vi "Build HW Tree.vi"(8 "error in (no error)":errorcluster, 10 "HW Info":T1[](array[typedef]), 11 "Hardware Info Module in":refnum<class "Hardware Info Module.lvclass">) -> (0 "error out":errorcluster, 3 "Hardware Info Module out":refnum<class "Hardware Info Module.lvclass">)   [LabVIEW 2023, in "Volatus.lvlib" / "Hardware Info Module.lvclass"]
uses:
  Hardware Info Module.lvclass
  HW Info.ctl
  lv-cdm/CDM-Config/Config-JSON/Config-JSON.lvclass
  Hardware Info Module.lvclass/Hardware Info Module.ctl
  lv-cdm/CDM-Config/Config Element/Config Element.lvclass
  lv-cdm/CDM-Config/Config Manager/Config Manager.lvclass
  <vilib>/JDP Science/JSONtext/JSONtext.lvlib
panel:
  out "JSON":string
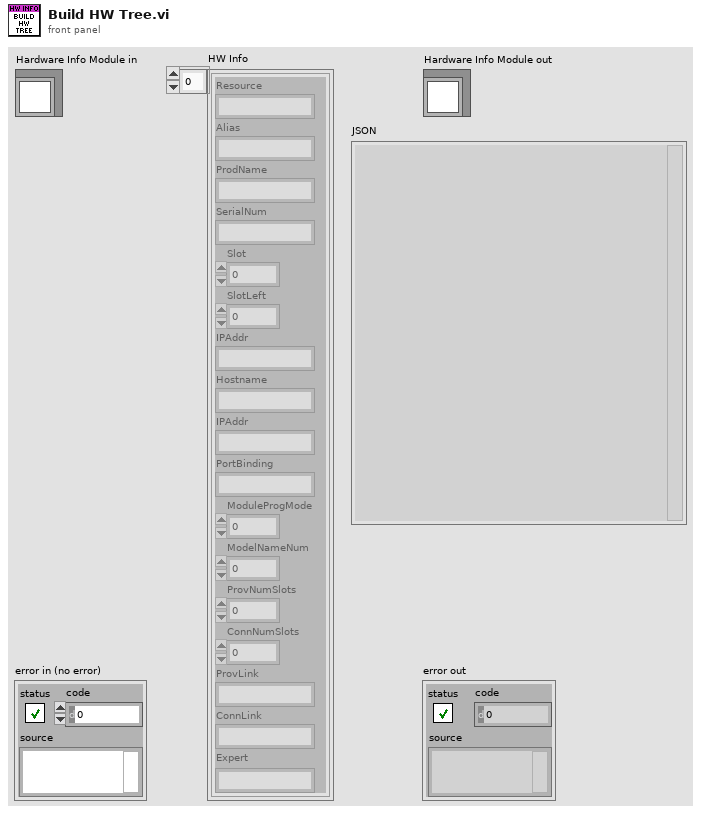
[diagram p1: front panel]
types:
  T1 = typedef "Volatus.lvlib/Hardware Info Module.lvclass/HW Info.ctl" = cluster{"Resource":string, "Alias":string, "ProdName":string, "SerialNum":string, "Slot":i32, "SlotLeft":u32, "IPAddr":string, "Hostname":string, "IPAddr":string, "PortBinding":string, "ModuleProgMode":u32, "ModelNameNum":u32, "ProvNumSlots":i32, "ConnNumSlots":i32, "ProvLink":string, "ConnLink":string, "Expert":string}
  T2 = typedef "Volatus.lvlib/Hardware Type.ctl" = enum16{"PC", "cRIO", "PXI"}
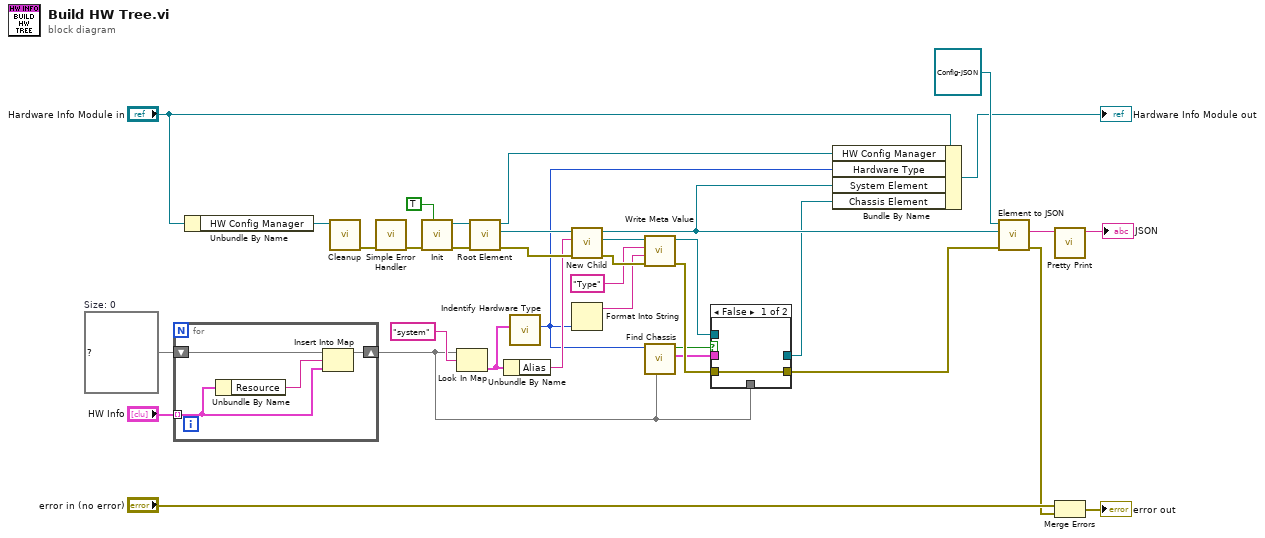
[diagram p0: block diagram]
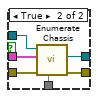
[diagram p2: hidden frame]
diagram:
  w31 = map{string, T1} {}  # Size: 0
  n1 = for {
    shift-right: [w36] -> w8
    shift-left: w31 -> [w39]
    tunnel: "HW Info" -> [w37] mode=indexing
    n2 = Unbundle By Name(w37) -> ("Resource"=w38:string)
    n3 = Insert Into Map(map in=w39, key=w38, value=w37) -> (map out=w36:map{string, T1})  [unwired: 2 out]
  }
  n4 = Unbundle By Name("Hardware Info Module in") -> ("HW Config Manager"=w27:refnum<class "Config Manager.lvclass">)
  n5 = call "Cleanup.vi"("Config Manager in"=w27) -> ("error out"=w26:errorcluster)  [unwired: 10 in]
  n6 = call <vilib>:"Simple Error Handler.vi"("error in (no error)"=w26) -> ("error out"=w25:errorcluster)  [unwired: 4 in, 4 out]
  n7 = call "Init.vi"("Mutable (F)"=TRUE ("Unlock Writes (F)"), "error in (no error)"=w25) -> ("error out"=w17:errorcluster, "Config Manager out"=w24:refnum<class "Config Manager.lvclass">)  [unwired: 8 in]
  n8 = Look In Map(map=w8, key="system") -> (value=w21:T1)  [unwired: 1 in, 1 out]
  n9 = call "Root Element.vi"("error in (no error)"=w17, "Config Manager in"=w24) -> ("error out"=w34:errorcluster, "Root Element"=w23:refnum<class "Config Element.lvclass">, "Config Manager out"=w5:refnum<class "Config Manager.lvclass">)  [unwired: 7 in]
  n10 = Unbundle By Name(w21) -> ("Alias"=w22:string)
  n11 = call "Indentify Hardware Type.vi"("Hw Info"=w21) -> ("Hardware Type"=w6:T2)  [unwired: 8 in, 2 out]
  n12 = call "New Child.vi"("error in (no error)"=w34, "Child Name"=w22, "Config Element in"=w23) -> ("error out"=w33:errorcluster, "New Child"=w20:refnum<class "Config Element.lvclass">, "Config Element out"=w10:refnum<class "Config Element.lvclass">)  [unwired: 6 in]
  n13 = Format Into String(w6) -> (resulting string=w19:string)  [unwired: 3 in, 1 out]
  n14 = call "Write Meta Value.vi"("error in (no error)"=w33, "Meta Value"=w19, "Meta Name"="Type", "Config Element in"=w20) -> ("error out"=w35:errorcluster, "Config Element out"=w2:refnum<class "Config Element.lvclass">)  [unwired: 6 in]
  n15 = call "Find Chassis.vi"("Map"=w8, "Hardware Type"=w6) -> ("Chassis Info"=w9:T1, "Has Chassis"=w7:bool)  [unwired: 8 in]
  n16 = case shown="False" w7 {
    tunnel: w35 -> [w40 w46]
    tunnel: w2 -> [_ w45]
    tunnel: w9 -> [_ w44]
    tunnel: w8 -> [_ w43]
    tunnel: [w40 w42] -> w3
    tunnel: [_ w41] -> w4
    frame False {
    }
    frame True {
      n17 = call "Enumerate Chassis.vi"("Map"=w43, "error in (no error)"=w46, "Chassis Info"=w44, "System Element"=w45) -> ("error out"=w42:errorcluster, "Chassis Element"=w41:refnum<class "Config Element.lvclass">)  [unwired: 6 in]
    }
  }
  n18 = Bundle By Name(cluster="Hardware Info Module in", "HW Config Manager"=w5, "Hardware Type"=w6, "System Element"=w10, "Chassis Element"=w4) -> (→"Hardware Info Module out":refnum<class "Hardware Info Module.lvclass">)
  n19 = call "Element to JSON.vi"("error in (no error)"=w3, "Element"=w10, "Config-JSON"=refnum<class "Config-JSON.lvclass"> refnum) -> ("error out"=w13:errorcluster, "JSON"=w16:string)  [unwired: 7 in]
  n20 = call <vilib>:"Pretty Print.vi"("JSON"=w16) -> ("<JSON>"=→"JSON":string)  [unwired: 8 in, 2 out]
  n21 = Merge Errors("error in (no error)", w13) -> (→"error out":errorcluster)
